vi "SACB Loop.vi"(8 "error in":errorcluster, 11 "Notifier in":refnum<notifier>) -> (0 "error out":errorcluster, 3 "Notifier out":refnum<notifier>)   [LabVIEW 2017]
uses:
  controls/Model Name.ctl
  GV/All Inputs.vi
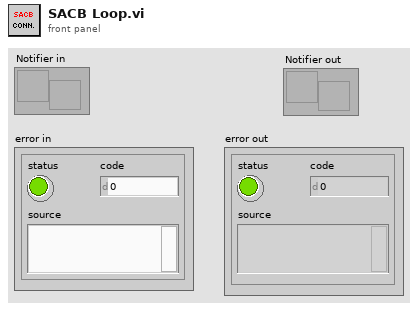
[diagram p1: front panel]
types:
  T1 = typedef "Model Name.ctl" = enum16{"W 501 FLH Std.", "W 501 FRH Std.", "W 601 FR RH Std", "W 601 FR LH Std", "W 601 RR RH Std", "W 601 RR LH Std", "W 601 FR RH AP", "W 601 FR LH AP", "W 601 RR RH AP", "W 601 RR LH AP"}
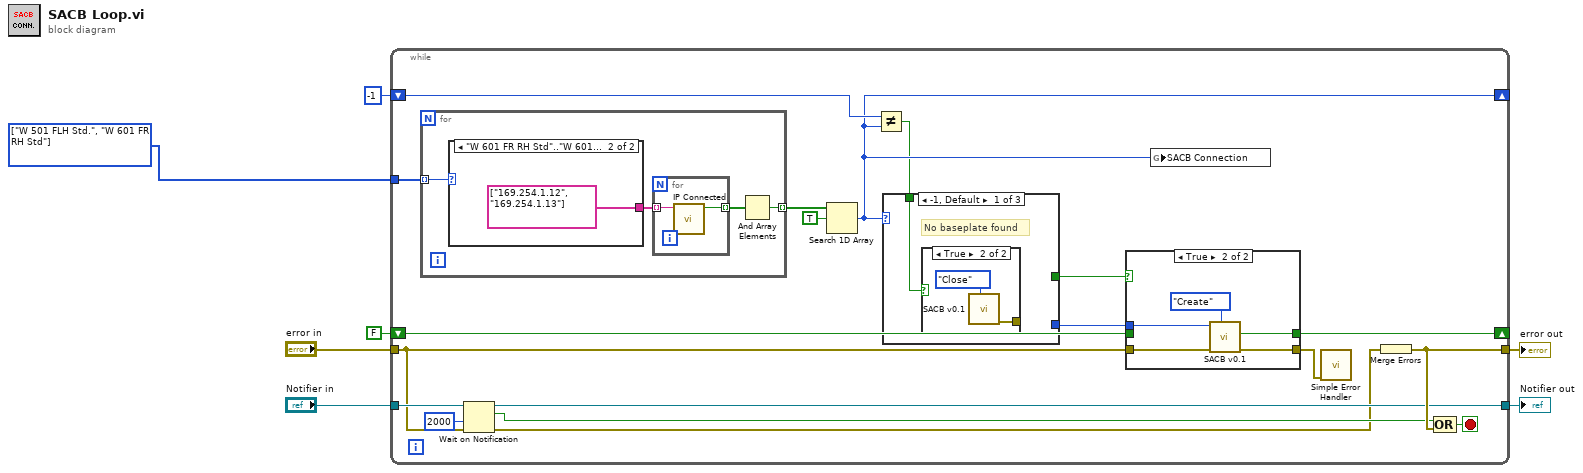
[diagram p0: block diagram]
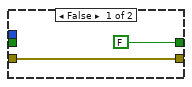
[diagram p2: hidden frame]
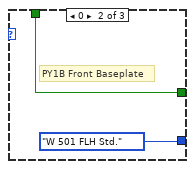
[diagram p4: hidden frame]
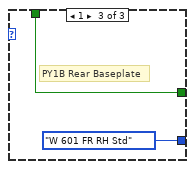
[diagram p5: hidden frame]
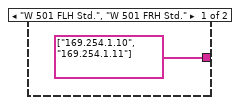
[diagram p6: hidden frame]
diagram:
  w1 = T1[] [enum."W 501 FLH Std.", enum."W 601 FR RH Std"] items=["W 501 FLH Std.", "W 501 FRH Std.", "W 601 FR RH Std", "W 601 FR LH Std", "W 601 RR RH Std", "W 601 RR LH Std", "W 601 FR RH AP", "W 601 FR LH AP", "W 601 RR RH AP", "W 601 RR LH AP"]
  n1 = while {
    tunnel: "error in" -> [w19]
    tunnel: [w25] -> w3
    tunnel: "Notifier in" -> [w24]
    tunnel: [w21] -> w6
    shift-right: [w14] -> _
    shift-left: FALSE ("Connected?") -> [w13]
    shift-right: [w11] -> _
    shift-left: -1 ("index of element") -> [w12]
    tunnel: w1 -> [w8]
    stop <- w26 stop-if-true
    n2 = for {
      tunnel: [w42] -> w18 mode=indexing
      tunnel: w8 -> [w41] mode=indexing
      n3 = case shown="\"W 601 FR RH Std\"..\"W 601 RR LH AP\"" w41 {
        tunnel: [string[] ["169.254.1.10", "169.254.1.11"] string[] ["169.254.1.12", "169.254.1.13"]] -> w44
        frame "W 501 FLH Std.", "W 501 FRH Std." {
        }
        frame "W 601 FR RH Std".."W 601 RR LH AP" {
        }
      }
      n4 = for {
        tunnel: w44 -> [w46] mode=indexing
        tunnel: [w45] -> w43 mode=indexing
        n5 = call "IP Connected.vi"("IP Address to Ping"=w46) -> ("Connected"=w45:bool)  [unwired: 10 in]
      }
      n6 = And Array Elements(Boolean array=w43) -> (logical AND=w42:bool)
    }
    n7 = Wait on Notification(notifier=w24, timeout in ms (-1)=2000, error in (no error)=w19) -> (notifier out=w21:refnum<notifier>, notification=w22:bool, error out=w20:errorcluster)  [unwired: 1 in, 1 out]
    n8 = Search 1D Array(1D array=w18, element=TRUE) -> (index of element=w11:i32)  [unwired: 1 in]
    n9 = Not Equal?(x=w12, y=w11) -> (x != y?=w10:bool)
    n10 = case shown="-1, Default" w11 {
      tunnel: [_ Model_Name."W 501 FLH Std." ("Model Name") Model_Name."W 601 FR RH Std" ("Model Name")] -> w16
      tunnel: [_ w37 w40] -> w15
      tunnel: w10 -> [w34 w37 w40]
      frame -1, Default {
        # "No baseplate found"
        n11 = case shown="True" w34 {
          tunnel: [_ w35] -> _
          frame False {
          }
          frame True {
            n12 = call "SACB v0.1.vi"("Command"=enum16{"Create", "Read", "Close"}."Close") -> ("Error Out"=w35:errorcluster)  [unwired: 8 in, 2 out]
          }
        }
      }
      frame 0 {
        # "PY1B Front Baseplate"
      }
      frame 1 {
        # "PY1B Rear Baseplate"
      }
    }
    n13 = case shown="True" w15 {
      tunnel: w19 -> [w28 w33]
      tunnel: [w28 w32] -> w9
      tunnel: w16 -> [_ w31]
      tunnel: [FALSE ("Connected?") w30] -> w14
      tunnel: w13 -> [_ _]
      frame False {
      }
      frame True {
        n14 = call "SACB v0.1.vi"("Command"=enum16{"Create", "Read", "Close"}."Create", "Error In"=w33, "Model Name"=w31) -> ("Error Out"=w32:errorcluster, "Connected?"=w30:bool)  [unwired: 6 in, 1 out]
      }
    }
    n15 = global write "All Inputs.vi" "SACB Connection"(w11) -> ()
    n16 = call <vilib>:"Simple Error Handler.vi"("error in (no error)"=w9) -> ()  [unwired: 4 in, 5 out]
    n17 = Merge Errors(w20) -> (w25:errorcluster)
    n18 = Compound Arithmetic op=OR(w22, w25) -> (w26:bool)
  }
  "error out" <- w3
  "Notifier out" <- w6
